vi "TTLfunction_171213.vi"(9 "RegionClicked":i32, 10 "TTLArray":T1(array[cluster]), 11 "INPUT STRING":string caption="Rename the region") -> (0 "TTLActivation":i32, 1 "ActivationCritaria":i32, 2 "Activation":string="STAYING", 3 "ON-OFF":bool)   [LabVIEW 2016]
panel:
  out "ON/OFF":bool
  out "StayingSec":i32
  out "EnteringSec":i32
  out "Activation":string="STAYING"
  in  "Tab Control":enum32{"Page 1", "Page 2"}(tab)
  in  "Save":bool
  in  "CurrentFunction":bool
  in  "AddFunction":bool
  in  "FUNCITON TO THE REGION":bool caption="FUNCTION TO THE REGION-1"
  in  "CancelButton":bool
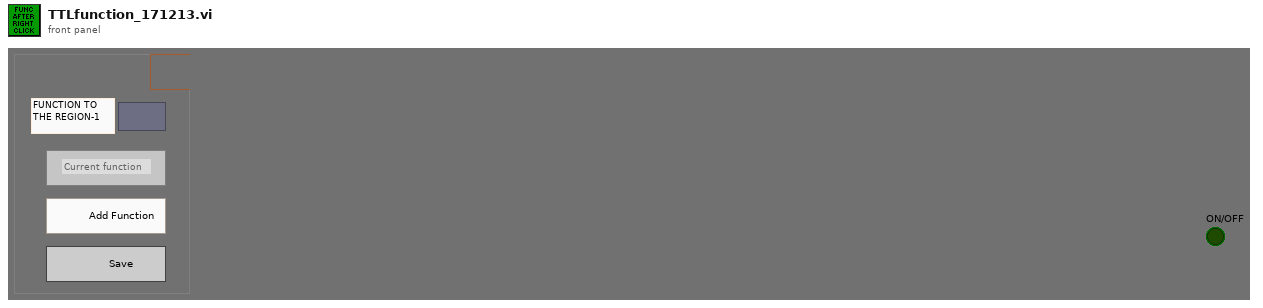
[diagram p1: front panel]
types:
  T1 = cluster{"Region number":i32, "ON/OFF":bool, "Activation type":string, "Activation critaria":i32, "Reward":i32}[]
  T2 = enum8{"Enabled", "Disabled", "Disabled and Grayed Out"}
  T3 = cluster{"Region number":i32, "ON/OFF":bool, "Activation type":string, "Activation critaria":i32, "Reward":i32}
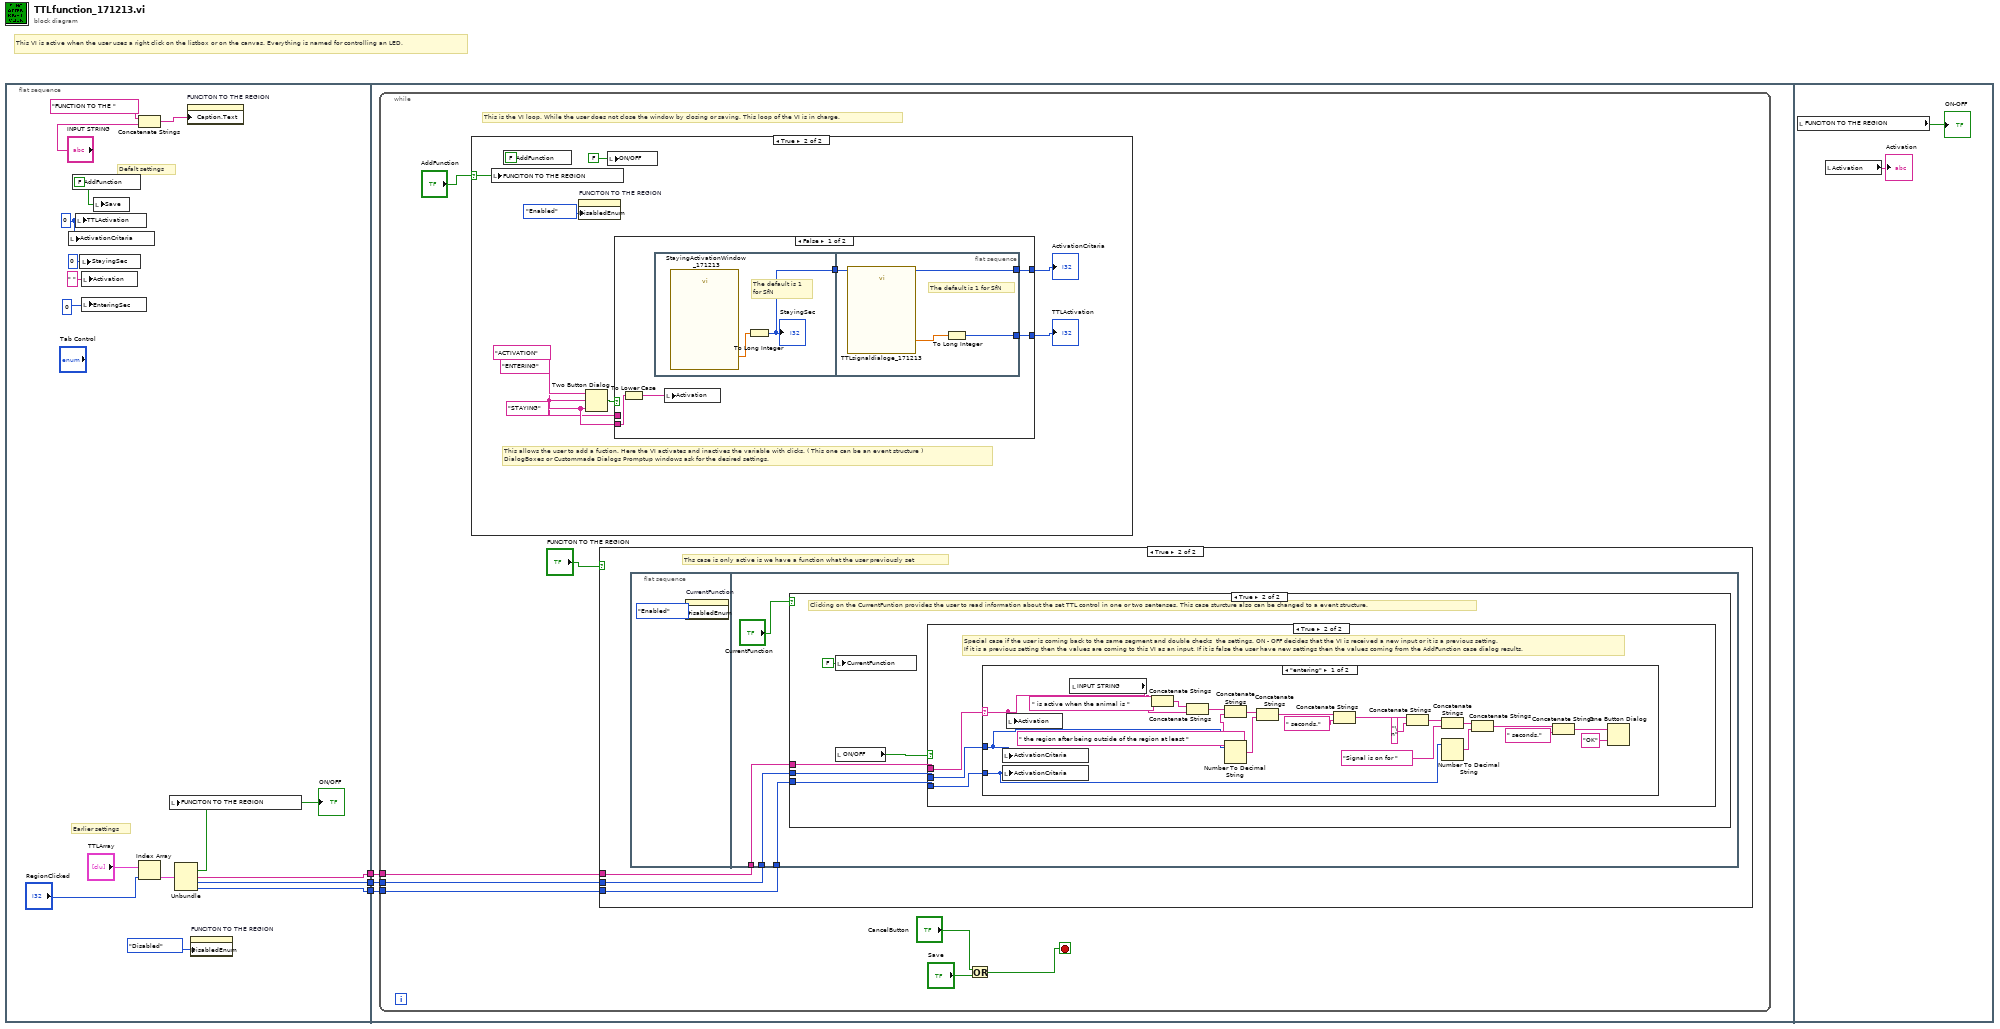
[diagram p0: block diagram]
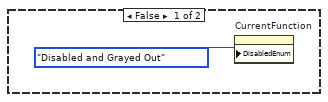
[diagram p2: hidden frame]
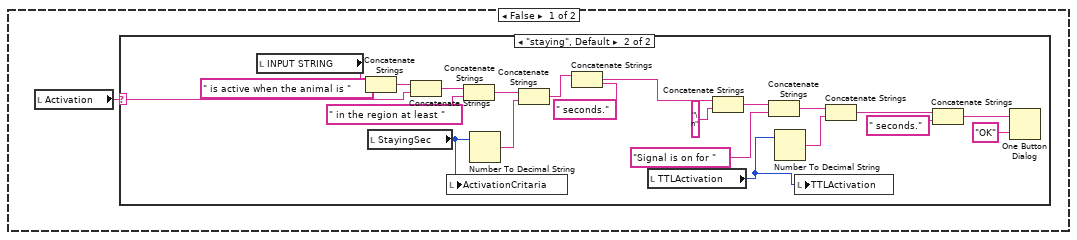
[diagram p4: hidden frame]
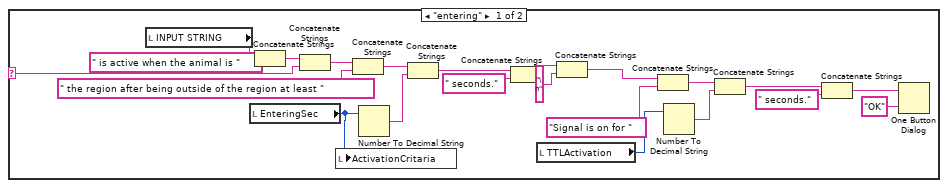
[diagram p5: hidden frame]
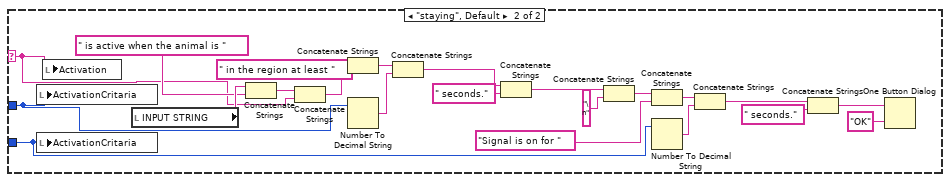
[diagram p6: hidden frame]
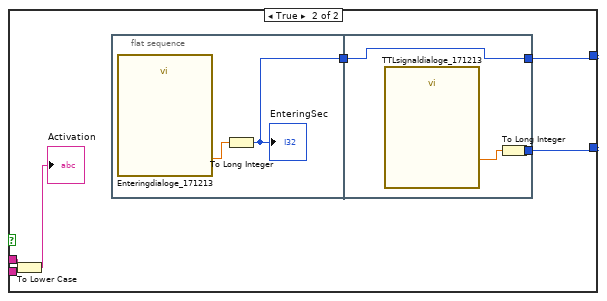
[diagram p8: hidden frame]
diagram:
  # "This VI is active when the user uses a right click on the listbox or on the canvas. Everything is named for controlling an LED."
  n1 = flat-sequence {
    tunnel: [w8] -> w3
    tunnel: [w7] -> w2
    tunnel: [w6] -> w1
    tunnel: w3 -> [w22]
    tunnel: w2 -> [w21]
    tunnel: w1 -> [w20]
    frame #0 {
      w13 = 0 ("Reward amount")
      w5 = FALSE ("add")
      # "Earlier settings"
      # "Defalt settings"
      n2 = local write "ActivationCritaria"(w13) -> ()
      n3 = local write "AddFunction"(w5) -> ()
      n4 = local write "TTLActivation"(w13) -> ()
      n5 = local write "StayingSec"(0 ("staying sec")) -> ()
      n6 = local write "Activation"(" " ("Activation")) -> ()
      n7 = local write "EnteringSec"(0 ("entering sec")) -> ()
      n8 = local write "Save"(w5) -> ()
      n9 = Concatenate Strings("FUNCTION TO THE " ("string"), "INPUT STRING") -> (w17:string)
      n10 = Index Array(array="TTLArray", index="RegionClicked") -> (element=w10:T3)
      n11 = Unbundle(w10) -> ("ON/OFF"=w9:bool, "Activation type"=w8:string, "Activation critaria"=w7:i32, "Reward"=w6:i32)  [unwired: 1 out]
      "ON/OFF" <- w9
      n12 = local write "FUNCITON TO THE REGION"(w9) -> ()
      n13 = property on="FUNCITON TO THE REGION" class="Bool (strict)"("Caption.Text"=w17) -> ()  [unwired: 2 in, 2 out]
      n14 = property on="FUNCITON TO THE REGION" class="Bool (strict)"("DisabledEnum"=T2."Disabled" ("Disabled")) -> ()  [unwired: 2 in, 2 out]
    }
    frame #1 {
      n15 = while {
        tunnel: w22 -> [w29]
        tunnel: w21 -> [w28]
        tunnel: w20 -> [w27]
        stop <- w24 stop-if-true
        # "This is the VI loop. While the user does not close the window by closing or saving. This loop of the VI is in charge."
        n16 = case shown="True" "AddFunction" {
          selector: "AddFunction" -> [_ w143]
          frame False {
          }
          frame True {
            w141 = "STAYING" ("F button name (\"Cancel\")")
            w140 = "ENTERING" ("T button name (\"OK\")")
            # "This allows the user to add a fuction. Here the VI activates and inactives the variable with clicks. ( This one can be an event structure ) \nDialogBoxes or Custommade Dialogs Promptup windows ask for the desired settings."
            n17 = local write "FUNCITON TO THE REGION"(w143) -> ()
            n18 = local write "AddFunction"(FALSE ("add")) -> ()
            n19 = property on="FUNCITON TO THE REGION" class="Bool (strict)"("DisabledEnum"=T2."Enabled" ("Disabled")) -> ()  [unwired: 2 in, 2 out]
            n20 = Two Button Dialog(message="ACTIVATION", 1:w141, 2:w140) -> (T button?=w145:bool)
            n21 = local write "ON/OFF"(FALSE ("ON/OFF")) -> ()
            n22 = case shown="False" w145 {
              tunnel: w141 -> [w150 _]
              tunnel: w140 -> [_ w160]
              tunnel: [w149 w159] -> w138
              tunnel: [w147 w157] -> w139
              frame False {
                n23 = To Lower Case(string=w150) -> (all lower case string=w151:string)
                n24 = flat-sequence {
                  tunnel: [w152] -> w148
                  tunnel: [w156] -> w149
                  tunnel: w148 -> [w156]
                  tunnel: [w154] -> w147
                  frame #0 {
                    # "The default is 1 \nfor SfN"
                    n25 = call "StayingActivationWindow_171213.vi"() -> ("(in seconds)"=w153:dbl)  [unwired: 17 in, 2 out]
                    n26 = To Long Integer(number=w153) -> (32bit integer=w152:i32)
                    "StayingSec" <- w152
                  }
                  frame #1 {
                    # "The default is 1 for SfN"
                    n27 = call "TTLsignaldialoge_171213.vi"() -> ("(in microliter)"=w155:dbl)  [unwired: 17 in, 2 out]
                    n28 = To Long Integer(number=w155) -> (32bit integer=w154:i32)
                  }
                }
                n29 = local write "Activation"(w151) -> ()
              }
              frame True {
                n30 = To Lower Case(string=w160) -> (all lower case string=→"Activation":string)
                n31 = flat-sequence {
                  tunnel: [w162] -> w158
                  tunnel: [w166] -> w159
                  tunnel: w158 -> [w166]
                  tunnel: [w165] -> w157
                  frame #0 {
                    n32 = call "Enteringdialoge_171213.vi"() -> ("(in seconds)"=w163:dbl)  [unwired: 17 in, 2 out]
                    n33 = To Long Integer(number=w163) -> (32bit integer=w162:i32)
                    "EnteringSec" <- w162
                  }
                  frame #1 {
                    n34 = call "TTLsignaldialoge_171213.vi"() -> ("(in microliter)"=w164:dbl)  [unwired: 17 in, 2 out]
                    n35 = To Long Integer(number=w164) -> (32bit integer=w165:i32)
                  }
                }
              }
            }
            "TTLActivation" <- w139
            "ActivationCritaria" <- w138
          }
        }
        n36 = case shown="True" "FUNCITON TO THE REGION" {
          tunnel: w29 -> [_ w34]
          tunnel: w28 -> [_ w33]
          tunnel: w27 -> [_ w32]
          frame False {
            n37 = property on="CurrentFunction" class="Bool (strict)"("DisabledEnum"=T2."Disabled and Grayed Out" ("Disabled")) -> ()  [unwired: 2 in, 2 out]
          }
          frame True {
            # "Ths case is only active is we have a function what the user previously set"
            n38 = flat-sequence {
              tunnel: w34 -> [w38]
              tunnel: w33 -> [w37]
              tunnel: w32 -> [w36]
              frame #0 {
                n39 = property on="CurrentFunction" class="Bool (strict)"("DisabledEnum"=T2."Enabled" ("Disabled")) -> ()  [unwired: 2 in, 2 out]
              }
              frame #1 {
                n40 = case shown="True" "CurrentFunction" {
                  tunnel: w38 -> [_ w43]
                  tunnel: w37 -> [_ w42]
                  tunnel: w36 -> [_ w41]
                  frame False {
                  }
                  frame True {
                    # "Clicking on the CurrentFuntion provides the user to read information about the set TTL control in one or two sentenses. This case sturcture also can be changed to a event structure."
                    n41 = local write "CurrentFunction"(FALSE ("Current function")) -> ()
                    n42 = local read "ON/OFF"() -> (w40:bool)
                    n43 = case shown="True" w40 {
                      tunnel: w43 -> [_ w92]
                      tunnel: w42 -> [_ w91]
                      tunnel: w41 -> [_ w90]
                      frame False {
                        n44 = local read "Activation"() -> (w45:string)
                        n45 = case shown="\"staying\", Default" w45 {
                          selector: w45 -> [w66 w89]
                          frame "entering" {
                            n46 = local read "INPUT STRING"() -> (w63:string)
                            n47 = local read "EnteringSec"() -> (w46:i32)
                            n48 = Concatenate Strings(w63, " is active when the animal is " ("message")) -> (w64:string)
                            n49 = Concatenate Strings(w64, w66) -> (w62:string)
                            n50 = local write "ActivationCritaria"(w46) -> ()
                            n51 = Concatenate Strings(w62, " the region after being outside of the region at least " ("string")) -> (w60:string)
                            n52 = Number To Decimal String(number=w46) -> (decimal integer string=w57:string)  [unwired: 1 in]
                            n53 = Concatenate Strings(w60, w57) -> (w59:string)
                            n54 = Concatenate Strings(w59, " seconds." ("string")) -> (w56:string)
                            n55 = local read "TTLActivation"() -> (w52:i32)
                            n56 = Concatenate Strings(w56, "\n" ("string")) -> (w54:string)
                            n57 = Concatenate Strings(w54, "Signal is on for " ("string")) -> (w51:string)
                            n58 = Number To Decimal String(number=w52) -> (decimal integer string=w50:string)  [unwired: 1 in]
                            n59 = Concatenate Strings(w51, w50) -> (w49:string)
                            n60 = Concatenate Strings(w49, " seconds." ("string")) -> (w47:string)
                            n61 = One Button Dialog(message=w47, button name ("OK")="OK") -> ()  [unwired: 1 out]
                          }
                          frame "staying", Default {
                            n62 = local read "INPUT STRING"() -> (w87:string)
                            n63 = Concatenate Strings(w87, " is active when the animal is " ("message")) -> (w85:string)
                            n64 = local read "StayingSec"() -> (w69:i32)
                            n65 = Concatenate Strings(w85, w89) -> (w84:string)
                            n66 = local write "ActivationCritaria"(w69) -> ()
                            n67 = Concatenate Strings(w84, " in the region at least " ("string")) -> (w82:string)
                            n68 = Number To Decimal String(number=w69) -> (decimal integer string=w81:string)  [unwired: 1 in]
                            n69 = Concatenate Strings(w82, w81) -> (w80:string)
                            n70 = Concatenate Strings(w80, " seconds." ("string")) -> (w71:string)
                            n71 = local read "TTLActivation"() -> (w68:i32)
                            n72 = Concatenate Strings(w71, "\n" ("string")) -> (w77:string)
                            n73 = Concatenate Strings(w77, "Signal is on for " ("string")) -> (w75:string)
                            n74 = Number To Decimal String(number=w68) -> (decimal integer string=w74:string)  [unwired: 1 in]
                            n75 = local write "TTLActivation"(w68) -> ()
                            n76 = Concatenate Strings(w75, w74) -> (w73:string)
                            n77 = Concatenate Strings(w73, " seconds." ("string")) -> (w70:string)
                            n78 = One Button Dialog(message=w70, button name ("OK")="OK") -> ()  [unwired: 1 out]
                          }
                        }
                      }
                      frame True {
                        # "Special case if the user is coming back to the same segment and double checks  the settings. ON - OFF decides that the VI is received a new input or it is a previous setting. \nIf it is a previous setting then the values are coming to this VI as an input. If it is false the user have new settings then the values coming from the AddFunction case dialog results."
                        n79 = case shown="\"entering\"" w92 {
                          selector: w92 -> [w96 w116]
                          tunnel: w91 -> [w95 w117]
                          tunnel: w90 -> [w94 w118]
                          frame "entering" {
                            n80 = local write "ActivationCritaria"(w95) -> ()
                            n81 = local write "ActivationCritaria"(w94) -> ()
                            n82 = local write "Activation"(w96) -> ()
                            n83 = local read "INPUT STRING"() -> (w111:string)
                            n84 = Concatenate Strings(w111, " is active when the animal is " ("message")) -> (w112:string)
                            n85 = Concatenate Strings(w112, w96) -> (w110:string)
                            n86 = Concatenate Strings(w110, " the region after being outside of the region at least " ("string")) -> (w108:string)
                            n87 = Number To Decimal String(number=w95) -> (decimal integer string=w105:string)  [unwired: 1 in]
                            n88 = Concatenate Strings(w108, w105) -> (w107:string)
                            n89 = Concatenate Strings(w107, " seconds." ("string")) -> (w104:string)
                            n90 = Concatenate Strings(w104, "\n" ("string")) -> (w102:string)
                            n91 = Concatenate Strings(w102, "Signal is on for " ("string")) -> (w101:string)
                            n92 = Number To Decimal String(number=w94) -> (decimal integer string=w100:string)  [unwired: 1 in]
                            n93 = Concatenate Strings(w101, w100) -> (w99:string)
                            n94 = Concatenate Strings(w99, " seconds." ("string")) -> (w97:string)
                            n95 = One Button Dialog(message=w97, button name ("OK")="OK") -> ()  [unwired: 1 out]
                          }
                          frame "staying", Default {
                            n96 = local write "ActivationCritaria"(w117) -> ()
                            n97 = local write "ActivationCritaria"(w118) -> ()
                            n98 = local write "Activation"(w116) -> ()
                            n99 = local read "INPUT STRING"() -> (w135:string)
                            n100 = Concatenate Strings(w135, " is active when the animal is " ("message")) -> (w133:string)
                            n101 = Concatenate Strings(w133, w116) -> (w132:string)
                            n102 = Concatenate Strings(w132, " in the region at least " ("string")) -> (w130:string)
                            n103 = Number To Decimal String(number=w117) -> (decimal integer string=w129:string)  [unwired: 1 in]
                            n104 = Concatenate Strings(w130, w129) -> (w128:string)
                            n105 = Concatenate Strings(w128, " seconds." ("string")) -> (w120:string)
                            n106 = Concatenate Strings(w120, "\n" ("string")) -> (w125:string)
                            n107 = Concatenate Strings(w125, "Signal is on for " ("string")) -> (w124:string)
                            n108 = Number To Decimal String(number=w118) -> (decimal integer string=w123:string)  [unwired: 1 in]
                            n109 = Concatenate Strings(w124, w123) -> (w122:string)
                            n110 = Concatenate Strings(w122, " seconds." ("string")) -> (w119:string)
                            n111 = One Button Dialog(message=w119, button name ("OK")="OK") -> ()  [unwired: 1 out]
                          }
                        }
                      }
                    }
                  }
                }
              }
            }
          }
        }
        n112 = Or(x="CancelButton", y="Save") -> (x .or. y?=w24:bool)
      }
    }
    frame #2 {
      n113 = local read "FUNCITON TO THE REGION"() -> (→"ON-OFF":bool)
      n114 = local read "Activation"() -> (→"Activation":string)
    }
  }
